vi "SelectAuton Path.vi"(8 "Scale":string, 9 "Switch":string, 11 "Auto Selector":string) -> (2 "What Auton to do":string)   [LabVIEW 2017]
panel:
  # "WeLeft"
  # "WeRight"
  # "WeCenter"
  # "Straight"
  # "None"
  # "Switch"
  # "SwitchOnly"
  # "SwitchOnly"
  # "PreferSwitch"
  # "PreferSwitch"
  # "PreferScale"
  # "PreferScale"
  # "ScaleOnly"
  # "ScaleOnly"
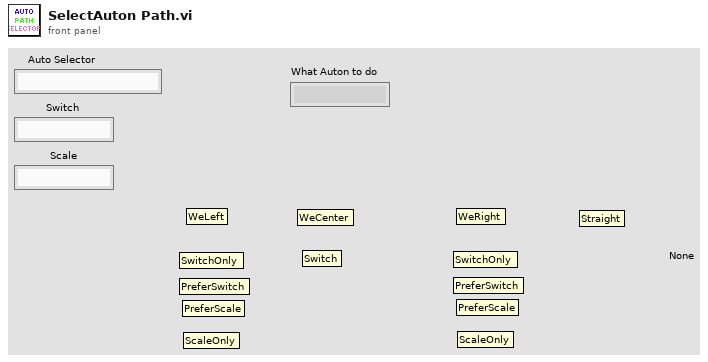
[diagram p1: front panel]
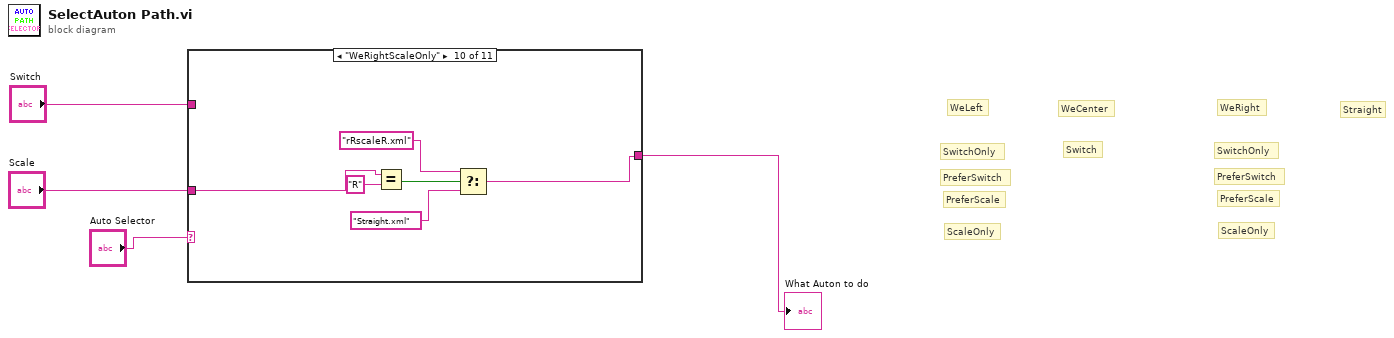
[diagram p0: block diagram]
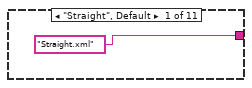
[diagram p2: hidden frame]
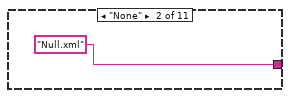
[diagram p3: hidden frame]
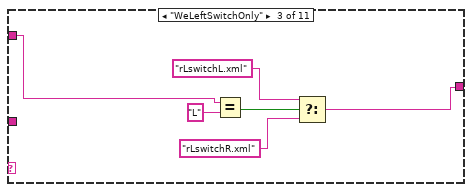
[diagram p4: hidden frame]
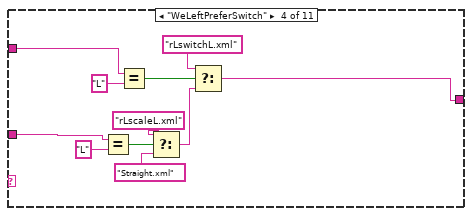
[diagram p5: hidden frame]
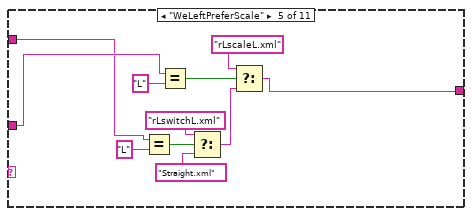
[diagram p6: hidden frame]
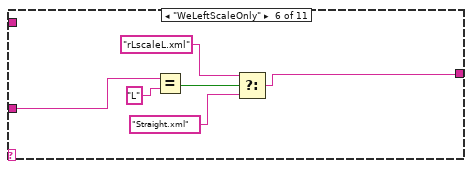
[diagram p7: hidden frame]
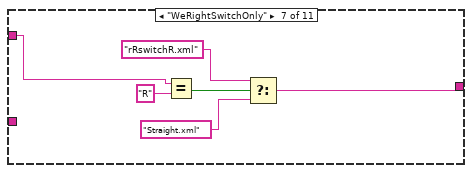
[diagram p8: hidden frame]
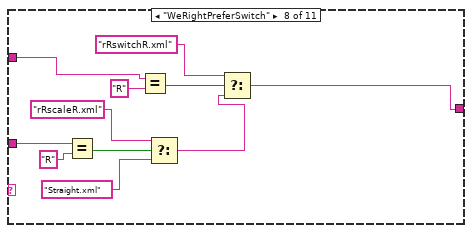
[diagram p9: hidden frame]
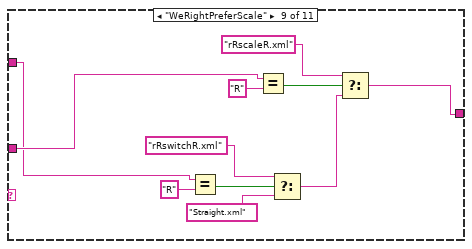
[diagram p10: hidden frame]
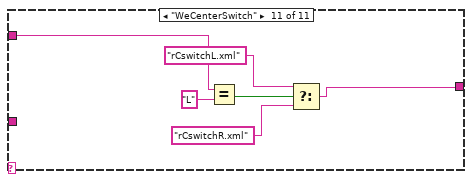
[diagram p11: hidden frame]
diagram:
  # "Straight"
  # "PreferScale"
  # "ScaleOnly"
  # "PreferSwitch"
  # "SwitchOnly"
  # "PreferScale"
  # "ScaleOnly"
  # "PreferSwitch"
  # "SwitchOnly"
  # "Switch"
  # "WeRight"
  # "WeCenter"
  # "WeLeft"
  n1 = case shown="\"WeRightScaleOnly\"" "Auto Selector" {
    tunnel: "Switch" -> [_ _ w8 w22 w24 _ w42 w54 w58 _ w80]
    tunnel: "Scale" -> [_ _ _ w20 w25 w36 _ w49 w65 w70 _]
    tunnel: ["Straight.xml" ("y") "Null.xml" ("y") w7 w13 w26 w35 w41 w47 w59 w69 w78] -> w1
    frame "Straight", Default {
    }
    frame "None" {
    }
    frame "WeLeftSwitchOnly" {
      n2 = Equal?(x=w8, y="L") -> (x = y?=w11:bool)
      n3 = Select(t="rLswitchL.xml" ("y"), s=w11, f="rLswitchR.xml" ("y")) -> (s? t:f=w7:string)
    }
    frame "WeLeftPreferSwitch" {
      n4 = Equal?(x=w20, y="L") -> (x = y?=w19:bool)
      n5 = Equal?(x=w22, y="L") -> (x = y?=w16:bool)
      n6 = Select(t="rLscaleL.xml" ("y"), s=w19, f="Straight.xml" ("y")) -> (s? t:f=w17:string)
      n7 = Select(t="rLswitchL.xml" ("y"), s=w16, f=w17) -> (s? t:f=w13:string)
    }
    frame "WeLeftPreferScale" {
      n8 = Equal?(x=w24, y="L") -> (x = y?=w32:bool)
      n9 = Equal?(x=w25, y="L") -> (x = y?=w29:bool)
      n10 = Select(t="rLswitchL.xml" ("y"), s=w32, f="Straight.xml" ("y")) -> (s? t:f=w30:string)
      n11 = Select(t="rLscaleL.xml" ("y"), s=w29, f=w30) -> (s? t:f=w26:string)
    }
    frame "WeLeftScaleOnly" {
      n12 = Equal?(x=w36, y="L") -> (x = y?=w39:bool)
      n13 = Select(t="rLscaleL.xml" ("y"), s=w39, f="Straight.xml" ("y")) -> (s? t:f=w35:string)
    }
    frame "WeRightSwitchOnly" {
      n14 = Equal?(x=w42, y="R") -> (x = y?=w45:bool)
      n15 = Select(t="rRswitchR.xml" ("y"), s=w45, f="Straight.xml" ("y")) -> (s? t:f=w41:string)
    }
    frame "WeRightPreferSwitch" {
      n16 = Equal?(x=w49, y="R") -> (x = y?=w52:bool)
      n17 = Equal?(x=w54, y="R") -> (x = y?=w56:bool)
      n18 = Select(t="rRscaleR.xml" ("y"), s=w52, f="Straight.xml" ("y")) -> (s? t:f=w48:string)
      n19 = Select(t="rRswitchR.xml" ("y"), s=w56, f=w48) -> (s? t:f=w47:string)
    }
    frame "WeRightPreferScale" {
      n20 = Equal?(x=w58, y="R") -> (x = y?=w63:bool)
      n21 = Equal?(x=w65, y="R") -> (x = y?=w67:bool)
      n22 = Select(t="rRswitchR.xml" ("y"), s=w63, f="Straight.xml" ("y")) -> (s? t:f=w60:string)
      n23 = Select(t="rRscaleR.xml" ("y"), s=w67, f=w60) -> (s? t:f=w59:string)
    }
    frame "WeRightScaleOnly" {
      n24 = Equal?(x=w70, y="R") -> (x = y?=w73:bool)
      n25 = Select(t="rRscaleR.xml" ("y"), s=w73, f="Straight.xml" ("y")) -> (s? t:f=w69:string)
    }
    frame "WeCenterSwitch" {
      n26 = Equal?(x=w80, y="L") -> (x = y?=w77:bool)
      n27 = Select(t="rCswitchL.xml" ("y"), s=w77, f="rCswitchR.xml" ("y")) -> (s? t:f=w78:string)
    }
  }
  "What Auton to do" <- w1
